vi "Init Events.vi"(8 "error in (no error)":errorcluster, 11 "SequenceViewPanel in":refnum<class "SequenceViewPanel.lvclass">) -> (0 "error out":errorcluster, 3 "SequenceViewPanel out":refnum<class "SequenceViewPanel.lvclass">)   [LabVIEW 2020, in "TSnax UI.lvlib" / "SequenceViewPanel.lvclass"]
uses:
  SequenceViewPanel.lvclass
  Set SequenceFile Request.ctl
  TSnax/SequenceFile/SequenceFile.lvclass
  Set SequenceFile Response.ctl
  SequenceViewPanel.lvclass/SequenceViewPanel.ctl
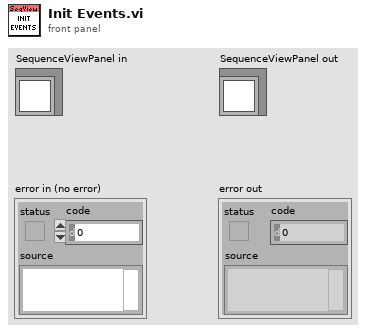
[diagram p1: front panel]
types:
  T1 = typedef "TSnax UI.lvlib/SequenceViewPanel.lvclass/Set SequenceFile Request.ctl" = cluster{"SequenceFile":refnum<class "SequenceFile.lvclass">, "Notifier":refnum<notifier>}
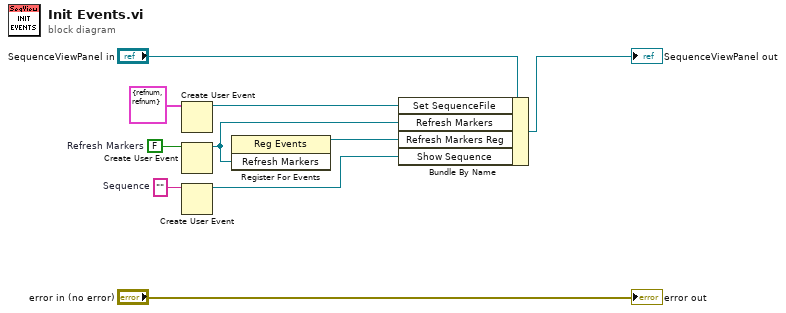
[diagram p0: block diagram]
diagram:
  w2 = ""  # Sequence
  w5 = FALSE  # Refresh Markers
  n1 = Create User Event(user event datatype=T1 {"SequenceFile"=refnum, "Notifier"=refnum} ("Set SequenceFile")) -> (user event=w6:refnum<user-event>)  [unwired: 1 in, 1 out]
  n2 = Create User Event(user event datatype=w5) -> (user event=w4:refnum<user-event>)  [unwired: 1 in, 1 out]
  n3 = Create User Event(user event datatype=w2) -> (user event=w1:refnum<user-event>)  [unwired: 1 in, 1 out]
  n4 = register-events(w4) -> (reference out=w3:refnum<event-registration>)  [unwired: 2 in, 1 out]
  n5 = Bundle By Name(cluster="SequenceViewPanel in", "Set SequenceFile"=w6, "Refresh Markers"=w4, "Refresh Markers Reg"=w3, "Show Sequence"=w1) -> (→"SequenceViewPanel out":refnum<class "SequenceViewPanel.lvclass">)
  "error out" <- "error in (no error)"
